vi "ReadData.vi"(8 "error in (no error)":errorcluster, 10 "timeout ms (100)":i32=100, 11 "reference in":refnum<class "NS master.lvclass">) -> (0 "error out":errorcluster, 1 "timed out?":bool, 2 "data":cdb[](array[numeric]), 3 "reference out":refnum<class "NS master.lvclass">)   [LabVIEW 2019, in "CommandResponse communication.lvlib" / "NS master.lvclass"]
doc: "Reads data streamed through data network stream"
uses:
  NS master.lvclass
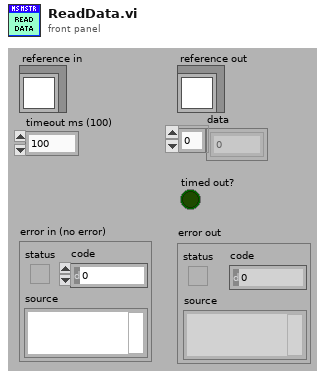
[diagram p1: front panel]
types:
  T1 = typedef "CommandResponse communication.lvlib/NS master.lvclass/ObjectAttributes.ctl" = cluster{"connected":bool, "stop":bool, "ID":string, "command wr":refnum<k21>, "response rd":refnum<k21>, "data rd":refnum<k21>, "slave ip":string, "slave id":string}
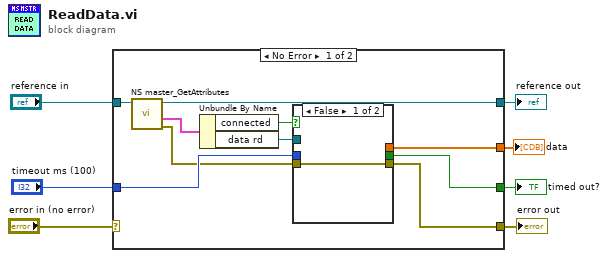
[diagram p0: block diagram]
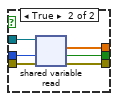
[diagram p2: hidden frame]
diagram:
  n1 = case shown="No Error" "error in (no error)" {
    selector: "error in (no error)" -> [_ w26]
    tunnel: [w9 w26] -> w6
    tunnel: [w17 w25] -> w4
    tunnel: "reference in" -> [w15 w25]
    tunnel: "timeout ms (100)" -> [w13 _]
    tunnel: [w12 _] -> w2
    tunnel: [w11 _] -> w1
    frame No Error {
      n2 = call "NS master_GetAttributes.vi"("reference in"=w15) -> ("error out"=w10:errorcluster, "attributes"=w16:T1, "reference out"=w17:refnum<class "NS master.lvclass">)  [unwired: 7 in, 1 out]
      n3 = Unbundle By Name(w16) -> ("connected"=w8:bool, "data rd"=w14:refnum<k21>)
      n4 = case shown="False" w8 {
        tunnel: w14 -> [_ w24]
        tunnel: w13 -> [_ w23]
        tunnel: [_ w22] -> w12
        tunnel: [_ w21] -> w11
        tunnel: w10 -> [w18 w20]
        tunnel: [w18 w19] -> w9
        frame False {
        }
        frame True {
          n5 = shared-variable-read(w24, w20, w23) -> (w19:errorcluster, w21:bool, w22:cdb[])  [unwired: 1 out]
        }
      }
    }
    frame Error {
    }
  }
  "error out" <- w6
  "reference out" <- w4
  "data" <- w2
  "timed out?" <- w1
